vi "Message.vi"(8 "error in (no error)":errorcluster, 10 "Message":string, 11 "Syslog_Event in":refnum<class "Event_Syslog.lvclass">) -> (0 "error out":errorcluster, 3 "Syslog_Event out":refnum<class "Event_Syslog.lvclass">)   [LabVIEW 2021, in "Event_Syslog.lvclass"]
uses:
  Event_Syslog.lvclass
  C:/Users/Tim/Documents/GitHub/Event_log/Source/abs_EventLog/abs_EventLog.lvclass
  abs_EventLog/abs_EventLog.lvclass/abs_EventLog.ctl
  Event_Syslog.lvclass/Event_Syslog.ctl
  abs_EventLog/Properties/Read Hostname.vi
  abs_EventLog/Properties/Read Message Tag.vi
  abs_EventLog/Properties/Read Facility Code.vi
  abs_EventLog/Properties/Read Severity Code.vi
  <vilib>/dlg_ctls.llb/Space Constant.vi
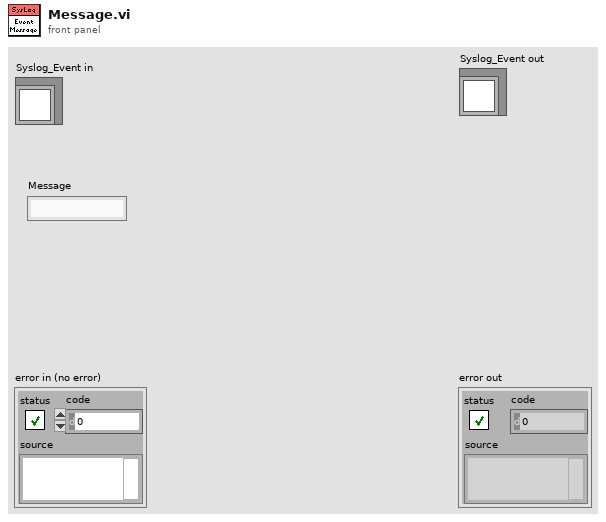
[diagram p1: front panel]
types:
  T1 = typedef "abs_EventLog.lvclass/Facility Code.ctl" = enum16{"kernel", "user", "mail", "system daemons", "security/authorization", "syslogd", "line printer", "network news", "uucp", "clock daemon", "security/authorization (alternate)", "FTP daemon", "NTP subsystem", "log audit", "log alert", "clock daemon (alternate)", "local use 0", "local use 1", "local use 2", "local use 3", "local use 4", "local use 5", "local use 6", "local use 7"}
  T2 = typedef "abs_EventLog.lvclass/Severity Code.ctl" = enum16{"emergency", "alert", "critical", "error", "warning", "notice", "info", "debug"}
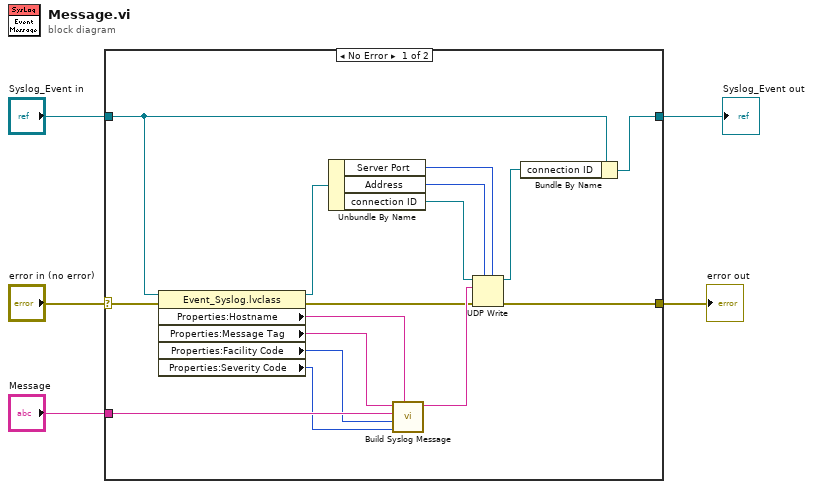
[diagram p0: block diagram]
diagram:
  n1 = case shown="No Error" "error in (no error)" {
    selector: "error in (no error)" -> [w13 w22]
    tunnel: [w18 w22] -> w5
    tunnel: [w16 w23] -> w4
    tunnel: "Message" -> [w14 _]
    tunnel: "Syslog_Event in" -> [w11 w23]
    frame No Error {
      n2 = property class="Event_Syslog.lvclass"(reference=w11, error in=w13) -> (reference out=w10:refnum<class "Event_Syslog.lvclass">, error out=w12:errorcluster, "Properties:Hostname"=w9:string, "Properties:Message Tag"=w8:string, "Properties:Facility Code"=w7:T1, "Properties:Severity Code"=w6:T2)
      n3 = Unbundle By Name(w10) -> ("Server Port"=w21:u16, "Address"=w20:u32, "connection ID"=w19:refnum<k16>)
      n4 = call "Build Syslog Message.vi"("Hostname"=w9, "Severity Code"=w6, "Facility Code"=w7, "Message Content"=w14, "Message Tag"=w8) -> ("Syslog Message"=w15:string)  [unwired: 6 in]
      n5 = UDP Write(address=w20, port or service name=w21, connection ID=w19, data in=w15, 8:w12) -> (error out=w18:errorcluster, 3:w17:refnum<k16>)  [unwired: 1 in]
      n6 = Bundle By Name(cluster=w11, "connection ID"=w17) -> (w16:refnum<class "Event_Syslog.lvclass">)
    }
    frame Error {
    }
  }
  "error out" <- w5
  "Syslog_Event out" <- w4
